vi "Spark API Example.vi"() -> ()   [LabVIEW 2014]
doc: "Simple example VI that uses the some of the Spark API to interact with a connected Spark device."
uses:
  Controls/Spark Reference.ctl
  <vilib>/httpClient/ClientHandle.ctl
  Controls/Device Query JSON.ctl
  Controls/Devices Query JSON.ctl
  Controls/Function Response JSON.ctl
  Spark API.lvlib
  <vilib>/httpClient/LabVIEWHTTPClient.lvlib
panel:
  out "A0 Value - Function Response":T1
  in  "stop":bool
  in  "Read A0":bool
  in  "Flash Tinker (Mac only)":bool
  in  "Get Current Spark Info":bool
  in  "Login to Spark Account":bool
  out "All Registered Spark Devices":T2
  in  "Spark Password":string
  in  "Spark Username":string
  out "error out":errorcluster
  out "Current Spark Reference Out":T3
  # "Run this VI and select the \"Login to Spark Account\" button, before choosing the other options."
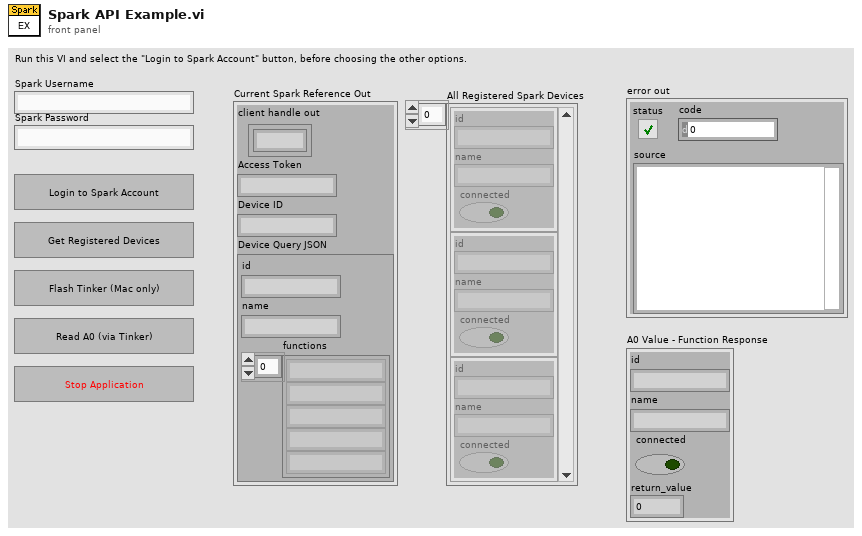
[diagram p1: front panel]
types:
  T1 = typedef "Spark API.lvlib/Function Response JSON.ctl" = cluster{"id":string, "name":string, "connected":bool, "return_value":dbl}
  T2 = typedef "Spark API.lvlib/Devices Query JSON.ctl" = cluster{"id":string, "name":string, "connected":bool}[]
  T3 = typedef "Spark API.lvlib/Spark Reference.ctl" = cluster{"client handle out":T4, "Access Token":string, "Device ID":string, "Device Query JSON":T5}
  T4 = typedef "LabVIEWHTTPClient.lvlib/ClientHandle.ctl" = refnum<k1>
  T5 = typedef "Spark API.lvlib/Device Query JSON.ctl" = cluster{"id":string, "name":string, "functions":string[]}
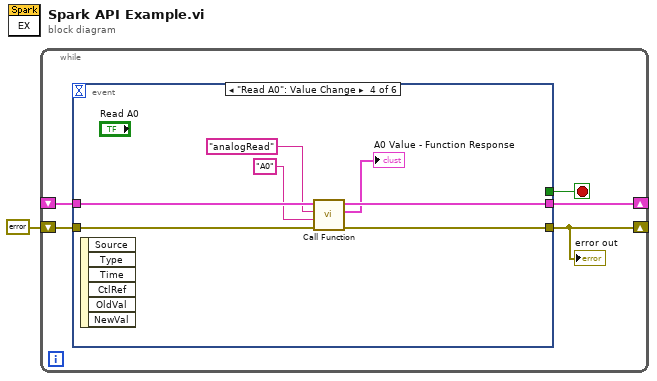
[diagram p0: block diagram]
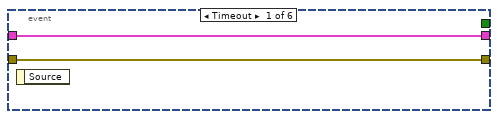
[diagram p2: hidden frame]
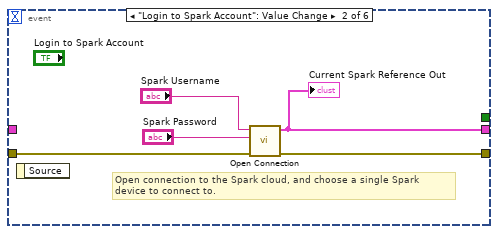
[diagram p3: hidden frame]
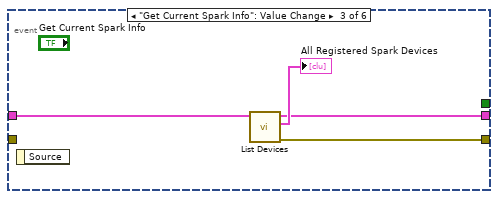
[diagram p4: hidden frame]
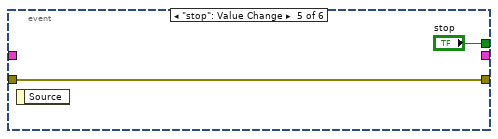
[diagram p5: hidden frame]
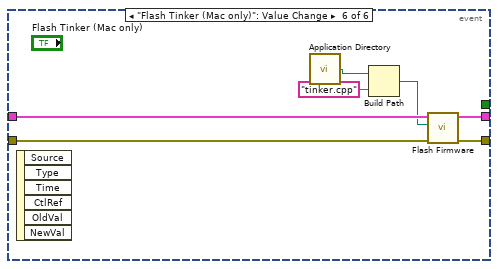
[diagram p6: hidden frame]
diagram:
  n1 = while {
    shift-right: [w6] -> _
    shift-left: _ -> [w5]
    shift-right: [w4] -> _
    shift-left: errorcluster {"status"=FALSE, "code"=0, "source"=""} ("error out") -> [w3]
    stop <- w2 stop-if-true
    n2 = event shown="[3] \"Read A0\": Value Change" {
      selector: _ -> [_ _ _ _ _ _]
      dyn-events: _ -> [_ _ _ _ _ _]
      timeout: _ -> [_ _ _ _ _ _]
      tunnel: [w7 w11 w15 w21 _ w30] -> w6
      tunnel: w5 -> [w7 _ w16 w24 _ w33]
      tunnel: [w8 w10 w14 w22 w26 w31] -> w4
      tunnel: w3 -> [w8 w9 _ w23 w26 w32]
      tunnel: [_ _ _ _ "stop" _] -> w2
      event Timeout {
        n3 = event-data() -> ()  [unwired: 1 in, 1 out]
      }
      event "Login to Spark Account": Value Change {
        # "Open connection to the Spark cloud, and choose a single Spark\ndevice to connect to."
        n4 = event-data() -> ()  [unwired: 1 in, 1 out]
        n5 = call "Open Connection.vi"("error in"=w9, "password"="Spark Password", "username"="Spark Username") -> ("error out"=w10:errorcluster, "Spark Reference"=w11:T3)  [unwired: 7 in]
        "Current Spark Reference Out" <- w11
      }
      event "Get Current Spark Info": Value Change {
        n6 = event-data() -> ()  [unwired: 1 in, 1 out]
        n7 = call "List Devices.vi"("Spark Reference In"=w16) -> ("error out"=w14:errorcluster, "Devices JSON"=→"All Registered Spark Devices":T2, "Spark Reference Out"=w15:T3)  [unwired: 8 in]
      }
      event "Read A0": Value Change {
        n8 = event-data() -> ()  [unwired: 1 in, 6 out]
        n9 = call "Call Function.vi"("error in"=w23, "Arguments"="A0", "Function Name"="analogRead", "Spark Reference In"=w24) -> ("error out"=w22:errorcluster, "Function Response"=→"A0 Value - Function Response":T1, "Spark Reference Out"=w21:T3)  [unwired: 5 in]
      }
      event "stop": Value Change {
        n10 = event-data() -> ()  [unwired: 1 in, 1 out]
      }
      event "Flash Tinker (Mac only)": Value Change {
        n11 = event-data() -> ()  [unwired: 1 in, 6 out]
        n12 = call <vilib>:"Application Directory.vi"() -> ("Application Directory"=w29:path)
        n13 = Build Path(base path=w29, name or relative path="tinker.cpp") -> (appended path=w27:path)
        n14 = call "Flash Firmware.vi"("error in"=w32, "Path to Code"=w27, "Spark Reference In"=w33) -> ("error out"=w31:errorcluster, "Spark Reference Out"=w30:T3)  [unwired: 7 in]
      }
    }
    "error out" <- w4
  }
